vi "485 to LEIN.vi"(7 "Header, data, CRC":u8[](array[numeric]), 11 "error in (no error)":errorcluster) -> (8 "CMD out":T1={"SID"=0, "ANF"=FALSE, "CMD"=enum."TASK", "DATA"=[]}, 10 "LEIN OK":bool, 15 "error out":errorcluster)   [LabVIEW 2011]
uses:
  Defenitions/LEIN CMD Cluster.ctl
  Defenitions/LEIN CMD List.ctl
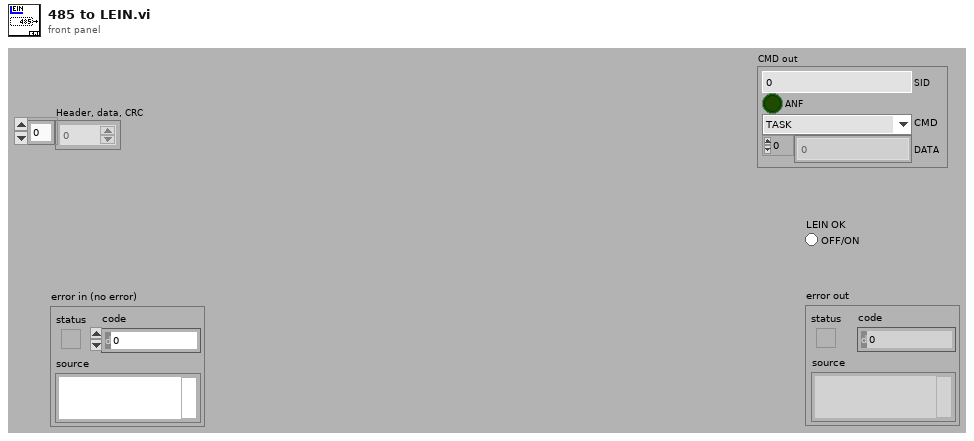
[diagram p1: front panel]
types:
  T1 = typedef "LEIN CMD Cluster.ctl" = cluster{"SID":u8, "ANF":bool, "CMD":T2, "DATA":u8[]}
  T2 = typedef "LEIN CMD List.ctl" = enum8{"ACTI", "TASK", "RES0", "STAT", "RES1", "RES2", "RES3", "USER"}
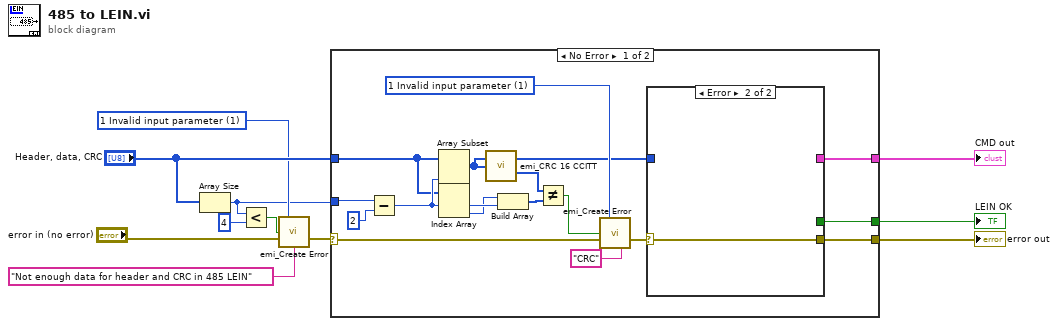
[diagram p0: block diagram]
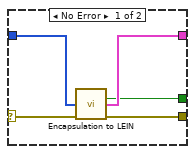
[diagram p2: hidden frame]
diagram:
  w5 = 1 items=["0 No Error"=0, "1 Invalid input parameter"=1, "6 Generic file IO "=6, "7 File not Found"=7, "35 Generic Pring Error"=35, "37 Device not Found"=37, "39 Device Unit Error"=39, "40 Could fot Open Device"=40, "42 Generic Error"=42, "52 Unknown Message"=52, "98 Bad File type"=98, "99 Bad File Version"=99, "100 Bad Data in File"=100, "1018 Unspecefied Error"=1018, "1041 Incorrect Password"=1041, "1043 Feature not in this version"=1043, "1109 Unsuported Data type"=1109, "1444 Did not close sucessfully"=1444] ("Error Code")
  n1 = Array Size(array="Header, data, CRC") -> (size(s)=w3:i32)
  n2 = Less?(x=w3, y=4) -> (x < y?=w8:bool)
  n3 = call "emi_Create Error.vi"("Error Code"=w5, "Error(T)"=w8, "error in (no error)"="error in (no error)", "Source String(\"\")"="Not enough data for header and CRC in 485 LEIN" ("Source String(\"\")")) -> ("error out"=w6:errorcluster)  [unwired: 11 in]
  n4 = case shown="No Error" w6 {
    selector: w6 -> [w20 w35]
    tunnel: [w28 w35] -> w11
    tunnel: "Header, data, CRC" -> [w22 _]
    tunnel: w3 -> [w27 _]
    tunnel: [w16 _] -> w2
    tunnel: [w14 _] -> w1
    frame No Error {
      w21 = 1 items=["0 No Error"=0, "1 Invalid input parameter"=1, "6 Generic file IO "=6, "7 File not Found"=7, "35 Generic Pring Error"=35, "37 Device not Found"=37, "39 Device Unit Error"=39, "40 Could fot Open Device"=40, "42 Generic Error"=42, "52 Unknown Message"=52, "98 Bad File type"=98, "99 Bad File Version"=99, "100 Bad Data in File"=100, "1018 Unspecefied Error"=1018, "1041 Incorrect Password"=1041, "1043 Feature not in this version"=1043, "1109 Unsuported Data type"=1109, "1444 Did not close sucessfully"=1444] ("Error Code")
      n5 = Subtract(x=w27, y=2) -> (x-y=w26:i32)
      n6 = Array Subset(array=w22, length=w26) -> (w17:u8[])  [unwired: 1 in]
      n7 = Index Array(array=w22, index #1=w26) -> (element #1=w24:u8, element #2=w12:u8)  [unwired: 1 in]
      n8 = call "emi_CRC 16 CCITT.vi"("Raw data"=w17) -> ("CCITT crc 16 bytes"=w23:u8[])  [unwired: 13 in, 1 out]
      n9 = Build Array(w12, w24) -> (w13:u8[])
      n10 = Not Equal?(x=w23, y=w13) -> (x != y?=w19:bool)
      n11 = call "emi_Create Error.vi"("Error Code"=w21, "Error(T)"=w19, "error in (no error)"=w20, "Append String(\"\")"="CRC" ("Append String(\"\")")) -> ("error out"=w18:errorcluster)  [unwired: 11 in]
      n12 = case shown="Error" w18 {
        selector: w18 -> [w32 w34]
        tunnel: [w33 w34] -> w28
        tunnel: w17 -> [w31 _]
        tunnel: [w30 _] -> w16
        tunnel: [w29 _] -> w14
        frame No Error {
          n13 = call "Encapsulation to LEIN.vi"("Data and header"=w31, "error in (no error)"=w32) -> ("LEIN OK"=w29:bool, "CMD out"=w30:T1, "error out"=w33:errorcluster)  [unwired: 10 in, 1 out]
        }
        frame Error {
        }
      }
    }
    frame Error {
    }
  }
  "error out" <- w11
  "CMD out" <- w2
  "LEIN OK" <- w1
